vi "PathPlanner_Cmd_AutoLTVUnicycleExecute.vi"(5 "PathPlanner_Cmd_FollowLTVUnicycleConfig":T18={"ControlPastEnd_Sec"=3.0, "Trigger Events"=TRUE, "LTV_Unicycle_Ctrl_Model"={"Max linear ctrl effort M/S"=2.0, "Max angular ctrl effort Rad/S"=0.7, "Max Heading Meas Tol Rad"=2.0, "Max X Pos Meas Tol M"=0.7, "Max Y Pos Meas Tol M"=0.7, "Max Linear Vel M/S"=2.0}, "X Tolerance M"=0.0762, "Y Tolerance M"=0.0762, "Rotation Tolerance DEG"=0.0872665, "Track Width Meters"=1.0, "Max Speed M/S"=4.0, "Period"=0.02} {"LTV_Unicycle_Ctrl_Model"."Max Linear Vel M/S" format="%#_13g"; "LTV_Unicycle_Ctrl_Model"."Max Y Pos Meas Tol M" format="%#_13g"; "LTV_Unicycle_Ctrl_Model"."Max X Pos Meas Tol M" format="%#_13g"; "LTV_Unicycle_Ctrl_Model"."Max Heading Meas Tol Rad" format="%#_13g"; "LTV_Unicycle_Ctrl_Model"."Max angular ctrl effort Rad/S" format="%#_13g"; "LTV_Unicycle_Ctrl_Model"."Max linear ctrl effort M/S" format="%#_13g"}, 6 "PassthroughTime_SEC":dbl=-1.0, 7 "PathPlanner_Cmd_AutoConfig":T3 {"Paths"."IdealStartingState"."Rotation"."SIN" format="%13.4f"; "Paths"."IdealStartingState"."Rotation"."COS" format="%13.4f"; "Paths"."IdealStartingState"."Rotation"."VALUE" format="%13.4f"; "Paths"."PointTowardsZones"."TargetPosition"."Y" format="%14.3f"; "Paths"."PointTowardsZones"."TargetPosition"."X" format="%14.3f"; "Paths"."PointTowardsZones"."RotationOffset"."SIN" format="%13.4f"; "Paths"."PointTowardsZones"."RotationOffset"."COS" format="%13.4f"; "Paths"."PointTowardsZones"."RotationOffset"."VALUE" format="%13.4f"; "Paths"."Waypoints"."nextControl"."Y" format="%14.3f"; "Paths"."Waypoints"."nextControl"."X" format="%14.3f"; "Paths"."Waypoints"."anchor"."Y" format="%14.3f"; "Paths"."Waypoints"."anchor"."X" format="%14.3f"; "Paths"."Waypoints"."prevControl"."Y" format="%14.3f"; "Paths"."Waypoints"."prevControl"."X" format="%14.3f"; "Paths"."AllPoints"."RotationTarget"."rotation"."SIN" format="%13.4f"; "Paths"."AllPoints"."RotationTarget"."rotation"."COS" format="%13.4f"; "Paths"."AllPoints"."RotationTarget"."rotation"."VALUE" format="%13.4f"; "Paths"."AllPoints"."Position"."Y" format="%14.3f"; "Paths"."AllPoints"."Position"."X" format="%14.3f"; "Paths"."GoalEndState"."Rotation"."SIN" format="%13.4f"; "Paths"."GoalEndState"."Rotation"."COS" format="%13.4f"; "Paths"."GoalEndState"."Rotation"."VALUE" format="%13.4f"; "Paths"."RotationTargets"."rotation"."SIN" format="%13.4f"; "Paths"."RotationTargets"."rotation"."COS" format="%13.4f"; "Paths"."RotationTargets"."rotation"."VALUE" format="%13.4f"}, 8 "Enabled":bool=TRUE, 9 "Reset":bool, 10 "CurrentChassisSpeeds":T2 {"vOmega" format="%10.3f"; "vY" format="%10.3f"; "vX" format="%10.3f"}, 11 "Current Pose SI":T20={"TRANSLATION"={"X"=0.0, "Y"=0.0}, "ROTATION"={"VALUE"=0.0, "COS"=1.0, "SIN"=0.0}} {"ROTATION"."SIN" format="%13.4f"; "ROTATION"."COS" format="%13.4f"; "ROTATION"."VALUE" format="%13.4f"; "TRANSLATION"."Y" format="%14.3f"; "TRANSLATION"."X" format="%14.3f"}) -> (0 "Position Error M":dbl, 1 "Complete":bool, 2 "At Reference":bool, 3 "Left Right Speed Dmds":T1)   [LabVIEW 2019, in "PathPlanner24.lvlib"]
doc: "DOCUMENTATION IS NOT COMPLETE.\n \nCalculates the next output of the path following controller for holonomic drive robots. This wraps a Holonomic Drive Control function with the particulars needed to follow a PathPlanner trajectory.\n\nInputs:\n - PathPlanner_Holonomic_Ctrl_Pack_Tuning - cluster - The tuning paraameters for the holonomic drive controller. These are static. They should not be changed after the first call to this function.\n - CurrentPoseSi - pose2d - The current pose calculated by odometry or pose estimation. The pose can be absolute or relative depending on what type of trajectory is being followed.\n - PathPlannerState - cluster - The path palnner trajectory state containing the desired position and velocities of the robot.\n - Reset - boolean - When TRUE the holonomic drive controller is reset. This should be set to TRUE for the first execution of a trajectory.\n - Enabled - boolean - When TRUE, closed loop control is enabled. (Optional. Default: TRUE)\n - Period - double - The loop period in seconds for this controller. (Optional. Default: 0.020)\n\nOutputs:\n - CalcChassisSpeed - cluster - The desired chassis speed in SI units.\n - AtReference - boolean - TRUE if the robots position is within the defined tolerance.\n - PositionError - pose2d - Position error in SI units. How far the robot is away from the desired trajectory position.\n - out_Holonomic_Drive_Ctrl - THe current holonomic drive controller data cluster. This is mainly for diagnostic purposes."
uses:
  <vilib>/Rock Robotics/WPI/ThirdParty/JAS_Junk/TrajLib/TypeDef/POSE2D.ctl
  <vilib>/Rock Robotics/WPI/ThirdParty/JAS_Junk/TrajLib/TypeDef/TRANSLATION2D.ctl
  <vilib>/Rock Robotics/WPI/ThirdParty/JAS_Junk/TrajLib/TypeDef/ROTATION2D.ctl
  TypeDef/PathPlannerCmdPathPlannerAutoConfig.ctl
  TypeDef/PathPlannerCommandUtil.ctl
  ENum/PathPlanner_CommandUtilType_ENUM.ctl
  TypeDef/PathPlannerPath.ctl
  TypeDef/PathPlannerRotationTarget.ctl
  TypeDef/PathPlannerConstraintsZone.ctl
  TypeDef/PathPlannerPathConstraints.ctl
  TypeDef/PathPlannerEventMarker.ctl
  TypeDef/PathPlannerGoalEndState.ctl
  TypeDef/PathPlannerPathPoint.ctl
  TypeDef/PathPlannerWaypoint.ctl
  TypeDef/PathPlannerPointTowardsZone.ctl
  TypeDef/PathPlannerIdealStartingState.ctl
  <vilib>/Rock Robotics/WPI/ThirdParty/JAS_Junk/TrajLib/TypeDef/CHASSIS_SPEEDS.ctl
  <vilib>/Utility/semaphor.llb/Obtain Semaphore Reference.vi
  <vilib>/Rock Robotics/WPI/ThirdParty/JAS_Junk/TrajLib/Timer_Reset.vi
  PathPlanner24.lvlib
  <vilib>/Rock Robotics/WPI/ThirdParty/JAS_Junk/TrajLib/Trajectory_Library.lvlib
  <vilib>/Rock Robotics/WPI/ThirdParty/JAS_Junk/TrajLib/TypeDef/LTV_UNICYCLE_CONTROLLER_MODEL_PARAMS.CTL
  TypeDef/PathPlannerCmdFollowLTVUnicycleConfig.ctl
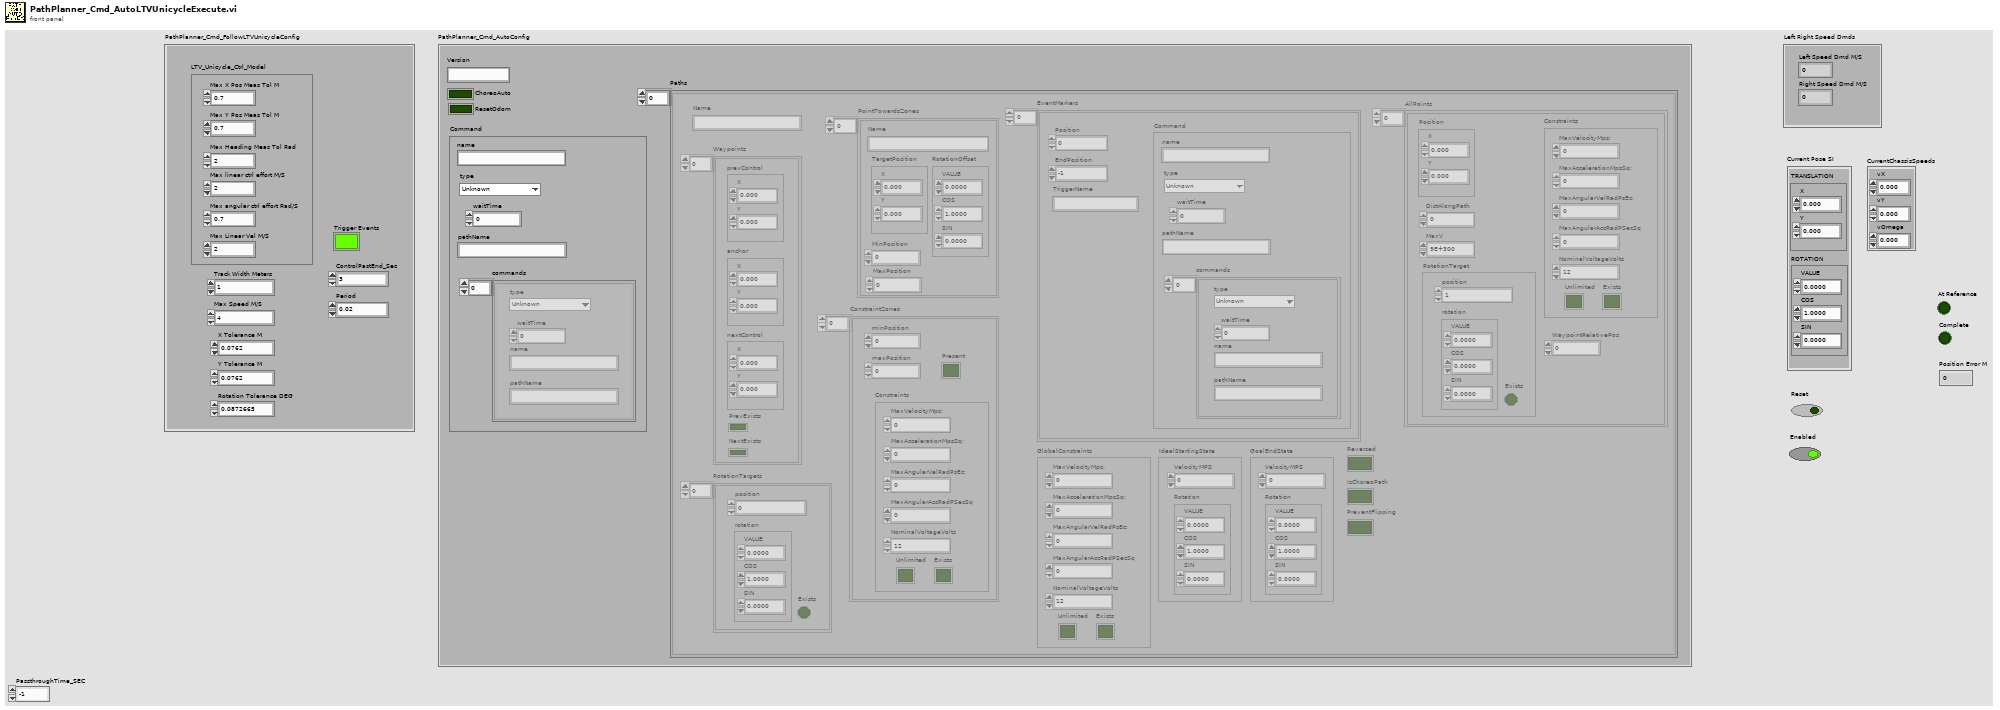
[diagram p1: front panel]
types:
  T1 = cluster{"Left Speed Dmd M/S":dbl, "Right Speed Dmd M/S":dbl}
  T2 = typedef "Trajectory_Library.lvlib/CHASSIS_SPEEDS.ctl" = cluster{"vX":dbl, "vY":dbl, "vOmega":dbl}
  T3 = typedef "PathPlanner24.lvlib/PathPlannerCmdPathPlannerAutoConfig.ctl" = cluster{"Command":T4, "ChoreoAuto":bool, "Version":string, "ResetOdom":bool, "Paths":T6[]}
  T4 = typedef "PathPlanner24.lvlib/PathPlannerCommandUtil.ctl" = cluster{"waitTime":dbl, "name":string, "pathName":string, "commands":cluster{"type":T5, "waitTime":dbl, "name":string, "pathName":string}[], "type":T5}
  T5 = typedef "PathPlanner24.lvlib/PathPlanner_CommandUtilType_ENUM.ctl" = enum16{"Unknown", "Wait", "Named", "Path", "Sequential", "Parallel", "Race", "Deadline"}
  T6 = typedef "PathPlanner24.lvlib/PathPlannerPath.ctl" = cluster{"Reversed":bool, "RotationTargets":T7[], "ConstraintZones":T9[], "EventMarkers":T11[], "GlobalConstraints":T10, "GoalEndState":T12, "AllPoints":T13[], "Name":string, "Waypoints":T15[], "PointTowardsZones":T16[], "IdealStartingState":T17, "IsChoreoPath":bool, "PreventFlipping":bool}
  T7 = typedef "PathPlanner24.lvlib/PathPlannerRotationTarget.ctl" = cluster{"position":dbl, "rotation":T8, "Exists":bool}
  T8 = typedef "Trajectory_Library.lvlib/ROTATION2D.ctl" = cluster{"VALUE":dbl, "COS":dbl, "SIN":dbl}
  T9 = typedef "PathPlanner24.lvlib/PathPlannerConstraintsZone.ctl" = cluster{"minPosition":dbl, "maxPosition":dbl, "Constraints":T10, "Present":bool}
  T10 = typedef "PathPlanner24.lvlib/PathPlannerPathConstraints.ctl" = cluster{"MaxVelocityMps;":dbl, "MaxAccelerationMpsSq;":dbl, "MaxAngularVelRadPsEc;":dbl, "MaxAngularAccRadPSecSq":dbl, "Exists":bool, "Unlimited":bool, "NominalVoltageVolts":dbl}
  T11 = typedef "PathPlanner24.lvlib/PathPlannerEventMarker.ctl" = cluster{"Position":dbl, "Command":T4, "TriggerName":string, "EndPosition":dbl}
  T12 = typedef "PathPlanner24.lvlib/PathPlannerGoalEndState.ctl" = cluster{"VelocityMPS":dbl, "Rotation":T8}
  T13 = typedef "PathPlanner24.lvlib/PathPlannerPathPoint.ctl" = cluster{"Position":T14, "DistAlongPath":dbl, "MaxV":dbl, "Constraints":T10, "RotationTarget":T7, "WaypointRelativePos":dbl}
  T14 = typedef "Trajectory_Library.lvlib/TRANSLATION2D.ctl" = cluster{"X":dbl, "Y":dbl}
  T15 = typedef "PathPlanner24.lvlib/PathPlannerWaypoint.ctl" = cluster{"prevControl":T14, "anchor":T14, "nextControl":T14, "PrevExists":bool, "NextExists":bool}
  T16 = typedef "PathPlanner24.lvlib/PathPlannerPointTowardsZone.ctl" = cluster{"RotationOffset":T8, "Name":string, "TargetPosition":T14, "MinPosition":dbl, "MaxPosition":dbl}
  T17 = typedef "PathPlanner24.lvlib/PathPlannerIdealStartingState.ctl" = cluster{"VelocityMPS":dbl, "Rotation":T8}
  T18 = typedef "PathPlanner24.lvlib/PathPlannerCmdFollowLTVUnicycleConfig.ctl" = cluster{"ControlPastEnd_Sec":dbl, "Trigger Events":bool, "LTV_Unicycle_Ctrl_Model":T19, "X Tolerance M":dbl, "Y Tolerance M":dbl, "Rotation Tolerance DEG":dbl, "Track Width Meters":dbl, "Max Speed M/S":dbl, "Period":dbl}
  T19 = typedef "Trajectory_Library.lvlib/LTV_UNICYCLE_CONTROLLER_MODEL_PARAMS.CTL" = cluster{"Max linear ctrl effort M/S":dbl, "Max angular ctrl effort Rad/S":dbl, "Max Heading Meas Tol Rad":dbl, "Max X Pos Meas Tol M":dbl, "Max Y Pos Meas Tol M":dbl, "Max Linear Vel M/S":dbl}
  T20 = typedef "Trajectory_Library.lvlib/POSE2D.ctl" = cluster{"TRANSLATION":T14, "ROTATION":T8}
  T21 = typedef "Trajectory_Library.lvlib/TIMER.ctl" = cluster{"StartTime":dbl, "Accumulated TIme":dbl, "Running":bool, "semaphore":T22}
  T22 = typedef "Semaphore RefNum" = refnum<k1>
  T23 = cluster{"type":T5, "waitTime":dbl, "name":string, "pathName":string}[]
  T24 = cluster{"type":T5, "waitTime":dbl, "name":string, "pathName":string}
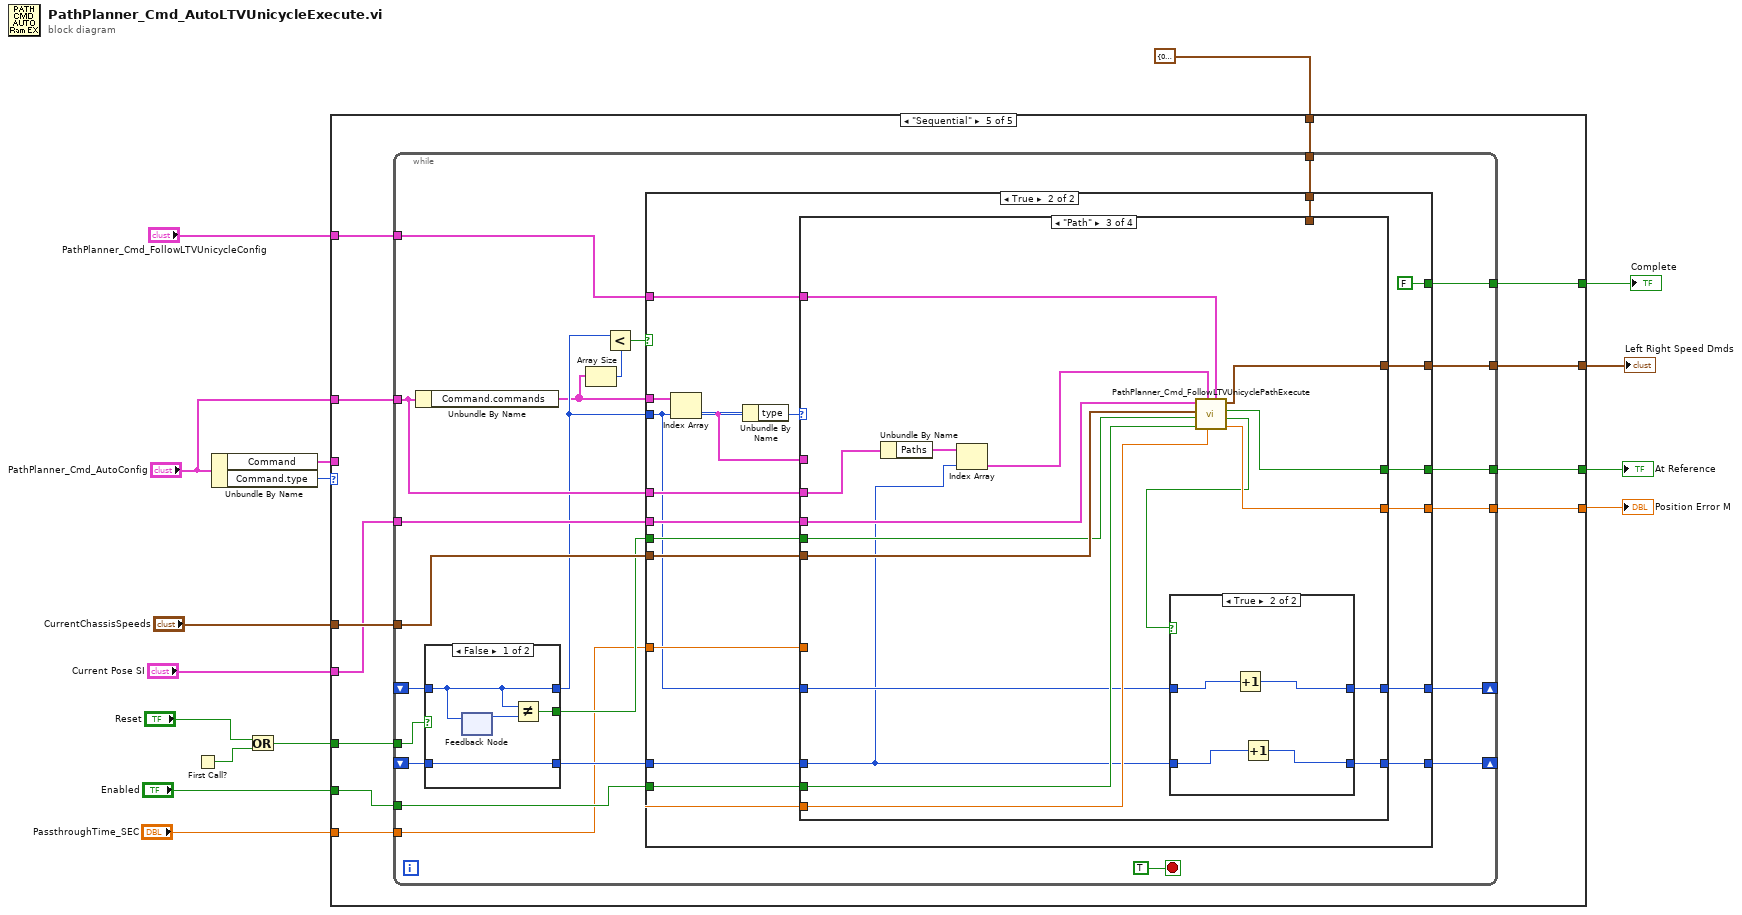
[diagram p0: block diagram]
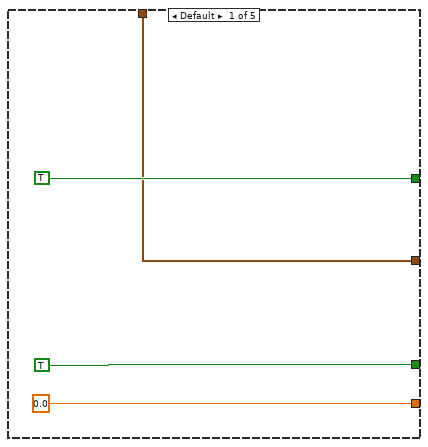
[diagram p2: hidden frame]
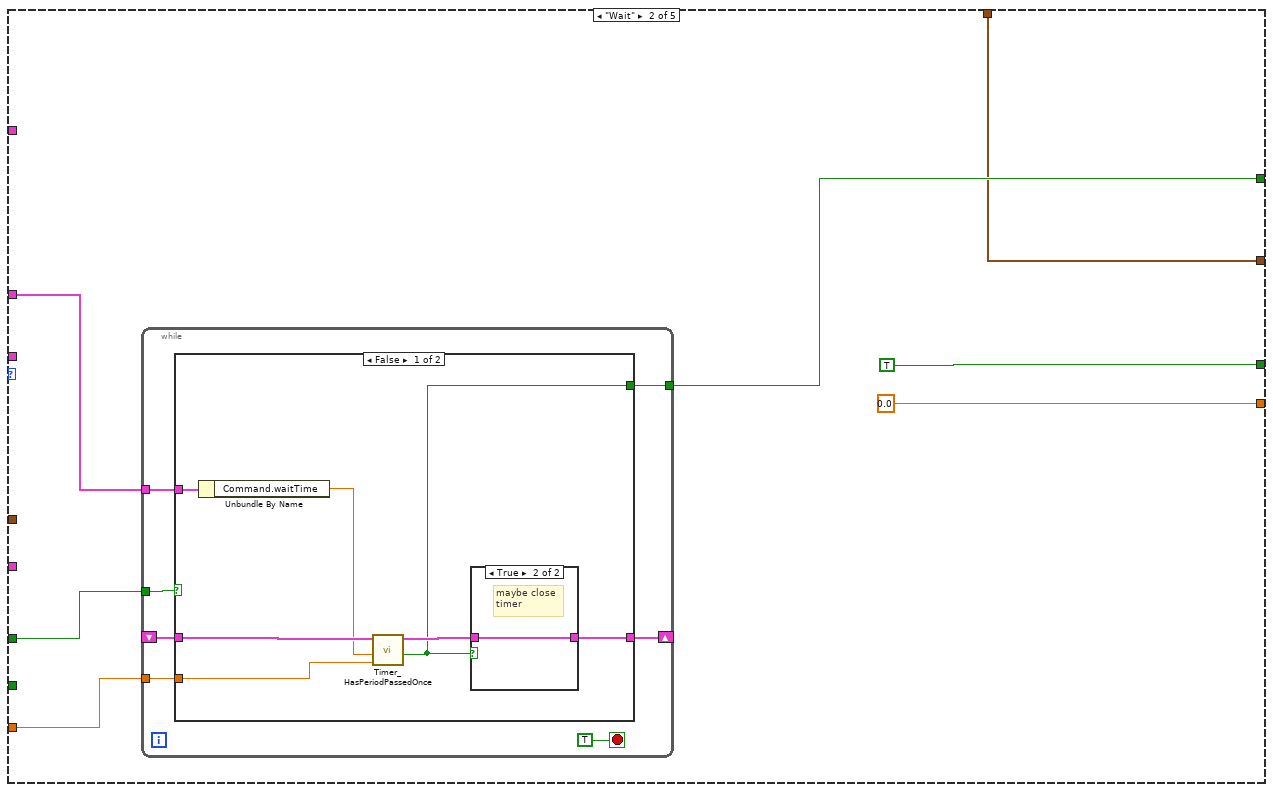
[diagram p3: hidden frame]
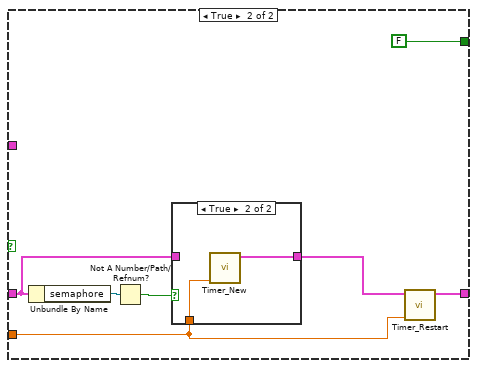
[diagram p5: hidden frame]
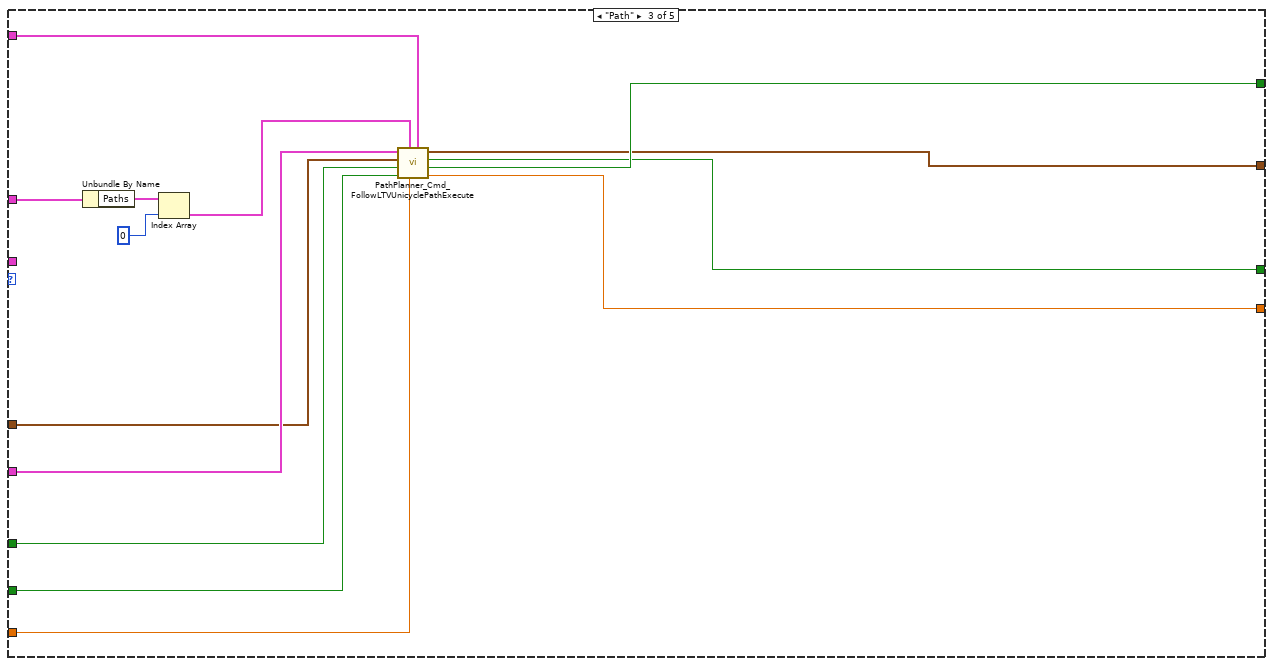
[diagram p7: hidden frame]
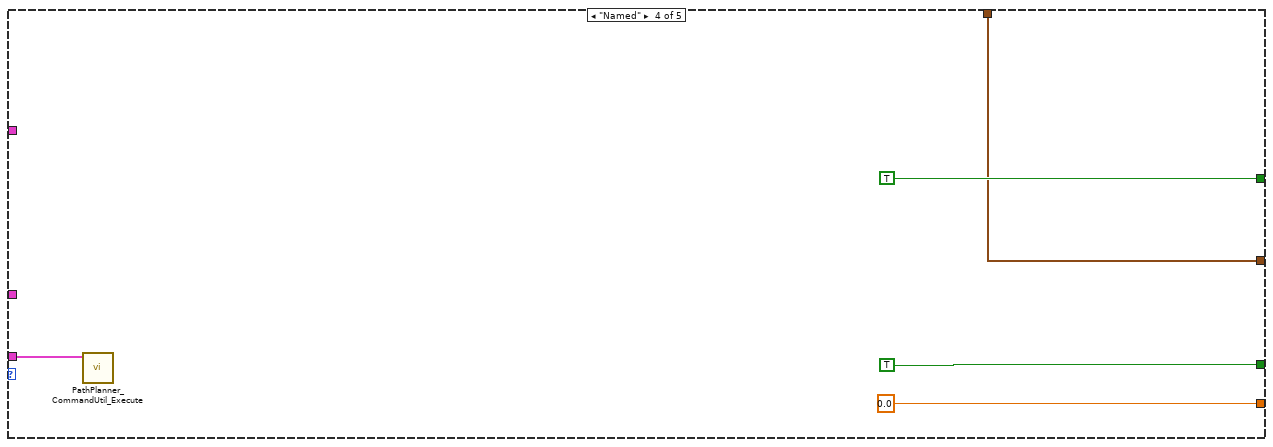
[diagram p8: hidden frame]
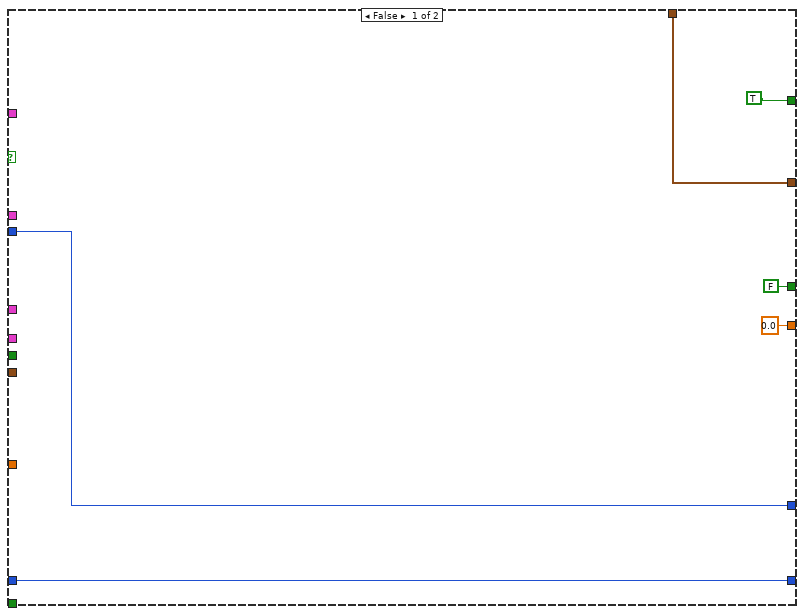
[diagram p9: hidden frame]
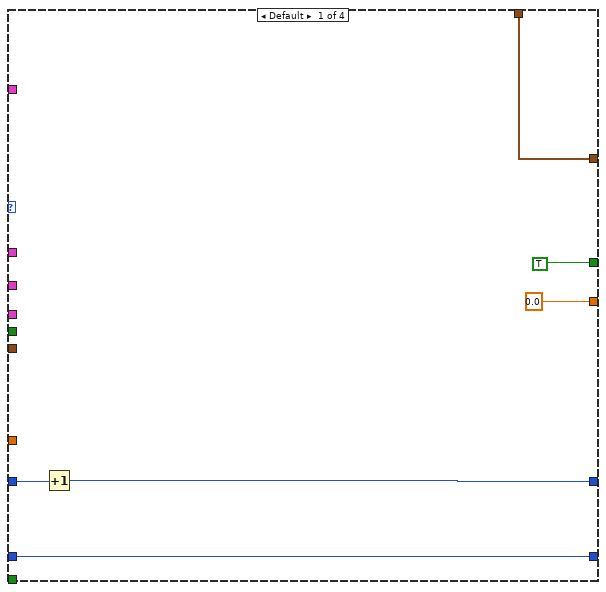
[diagram p10: hidden frame]
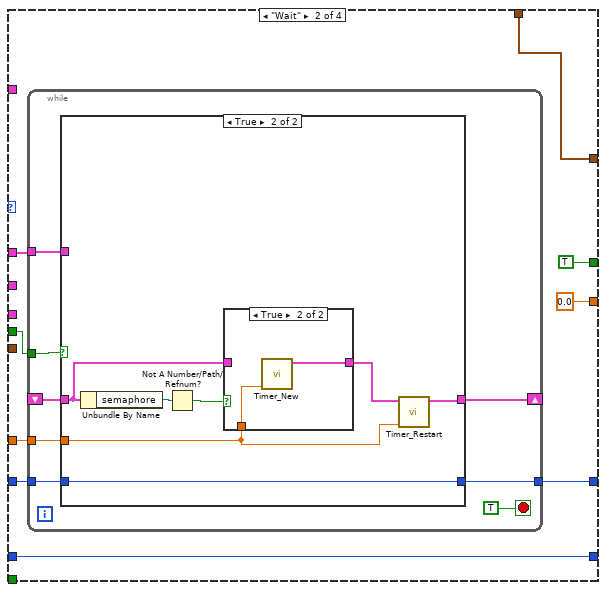
[diagram p11: hidden frame]
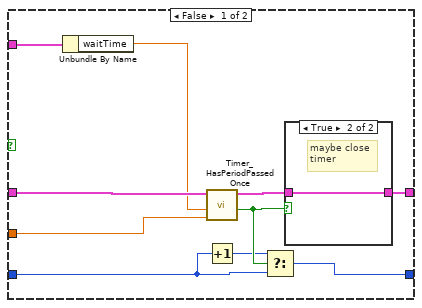
[diagram p12: hidden frame]
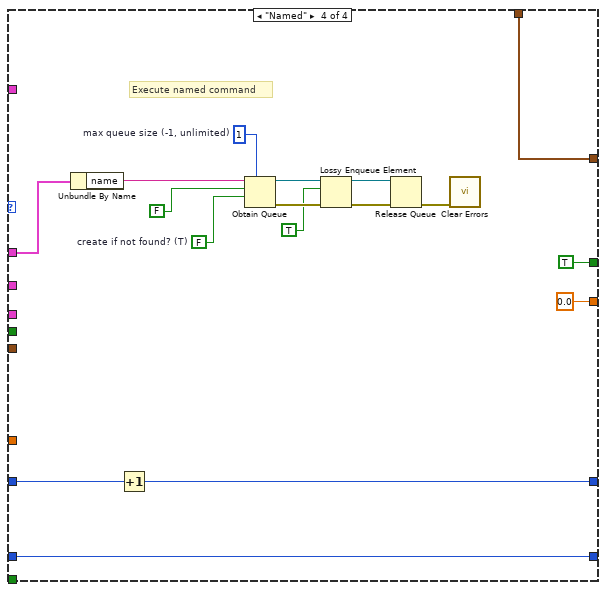
[diagram p16: hidden frame]
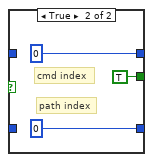
[diagram p17: hidden frame]
diagram:
  n1 = First Call?() -> (First Call?: T/F=w15:bool)
  n2 = Unbundle By Name("PathPlanner_Cmd_AutoConfig") -> ("Command"=w13:T4, "Command.type"=w14:T5)
  n3 = Or(x="Reset", y=w15) -> (x .or. y?=w8:bool)
  n4 = case shown="\"Sequential\"" w14 {
    tunnel: w13 -> [_ _ _ w72 _]
    tunnel: "PathPlanner_Cmd_AutoConfig" -> [_ w25 w67 _ w83]
    tunnel: "PathPlanner_Cmd_FollowLTVUnicycleConfig" -> [_ _ w63 _ w77]
    tunnel: "Current Pose SI" -> [_ _ w62 _ w76]
    tunnel: "CurrentChassisSpeeds" -> [_ _ w61 _ w82]
    tunnel: w8 -> [_ w27 w60 _ w84]
    tunnel: "Enabled" -> [_ _ w59 _ w75]
    tunnel: "PassthroughTime_SEC" -> [_ w26 w58 _ w79]
    tunnel: [0.0 ("Position Error M") 0.0 ("Position Error M") w57 0.0 ("Position Error M") w80] -> w5
    tunnel: [TRUE ("Complete") w24 w56 TRUE ("Complete") w74] -> w4
    tunnel: [TRUE ("At Reference") TRUE ("At Reference") w55 TRUE ("At Reference") w81] -> w3
    tunnel: T1 {"Left Speed Dmd M/S"=0.0, "Right Speed Dmd M/S"=0.0} ("Left Right Speed Dmds") -> [w17 w21 _ w68 w78]
    tunnel: [w17 w21 w54 w68 w73] -> w2
    frame Default {
    }
    frame "Wait" {
      n5 = while {
        tunnel: w27 -> [w34]
        tunnel: w26 -> [w33]
        shift-right: [w32] -> _
        shift-left: _ -> [w31]
        tunnel: w25 -> [w30]
        tunnel: [w28] -> w24
        stop <- TRUE stop-if-true
        n6 = case shown="False" w34 {
          tunnel: w33 -> [w40 w49]
          tunnel: [w36 w48] -> w32
          tunnel: w31 -> [w41 w44]
          tunnel: w30 -> [w39 _]
          tunnel: [w35 FALSE ("Expired")] -> w28
          frame False {
            n7 = Unbundle By Name(w39) -> ("Command.waitTime"=w38:dbl)
            n8 = call <vilib>:"Timer_HasPeriodPassedOnce.vi"("Pass_Through_Time"=w40, "Period"=w38, "in Timer"=w41) -> ("Expired"=w35:bool, "out Timer"=w37:T21)  [unwired: 6 in, 1 out]
            n9 = case shown="True" w35 {
              tunnel: w37 -> [w42 w43]
              tunnel: [w42 w43] -> w36
              frame False {
              }
              frame True {
                # "maybe close\ntimer"
              }
            }
          }
          frame True {
            n10 = Unbundle By Name(w44) -> ("semaphore"=w45:T22)
            n11 = Not A Number/Path/Refnum?(number/path/refnum=w45) -> (NaN/Path/Refnum?=w46:bool)
            n12 = case shown="True" w46 {
              tunnel: [w51 w53] -> w50
              tunnel: w49 -> [_ w52]
              tunnel: w44 -> [w51 _]
              frame False {
              }
              frame True {
                n13 = call <vilib>:"Timer_New.vi"("Pass_Through_Time"=w52) -> ("TIMER"=w53:T21)  [unwired: 10 in]
              }
            }
            n14 = call <vilib>:"Timer_Restart.vi"("Pass_Through_Time"=w49, "in Timer"=w50) -> ("out Timer"=w48:T21)  [unwired: 9 in]
          }
        }
      }
    }
    frame "Path" {
      n15 = Unbundle By Name(w67) -> ("Paths"=w66:T6[])
      n16 = Index Array(array=w66, index=0) -> (element=w64:T6)
      n17 = call "PathPlanner_Cmd_FollowLTVUnicyclePathExecute.vi"("PathPlanner_Cmd_FollowLTVUnicycleConfig"=w63, "PassthroughTime_SEC"=w58, "PathPlannerPath"=w64, "Enabled"=w59, "Reset"=w60, "CurrentChassisSpeeds"=w61, "Current Pose SI"=w62) -> ("Position Error M"=w57:dbl, "Complete"=w56:bool, "At Reference"=w55:bool, "Left Right Speed Dmds"=w54:T1)  [unwired: 1 out]
    }
    frame "Named" {
      n18 = call "PathPlanner_CommandUtil_Execute.vi"("Command"=w72) -> ()  [unwired: 11 in]
    }
    frame "Sequential" {
      n19 = while {
        tunnel: w84 -> [w103]
        tunnel: w83 -> [w98]
        tunnel: w82 -> [w106]
        tunnel: [w105] -> w81
        tunnel: [w104] -> w80
        tunnel: w79 -> [w93]
        shift-right: [w92] -> _
        shift-left: _ -> [w102]
        shift-right: [w91] -> _
        shift-left: _ -> [w101]
        tunnel: w78 -> [w99]
        tunnel: w77 -> [w96]
        tunnel: w76 -> [w95]
        tunnel: w75 -> [w94]
        tunnel: [w86] -> w74
        tunnel: [w85] -> w73
        stop <- TRUE stop-if-true
        n20 = Unbundle By Name(w98) -> ("Command.commands"=w88:T23)
        n21 = case shown="False" w103 {
          tunnel: [w218 0] -> w90
          tunnel: [w220 0] -> w97
          tunnel: w102 -> [w218 _]
          tunnel: w101 -> [w220 _]
          tunnel: [w221 TRUE] -> w100
          frame False {
            n22 = feedback-in #1(w218) -> ()
            n23 = feedback #1() -> (w219:i32)  [unwired: 1 in]
            n24 = Not Equal?(x=w218, y=w219) -> (x != y?=w221:bool)
          }
          frame True {
            # "path index"
            # "cmd index"
          }
        }
        n25 = Array Size(array=w88) -> (size(s)=w89:i32)
        n26 = Less?(x=w90, y=w89) -> (x < y?=w87:bool)
        n27 = case shown="True" w87 {
          tunnel: w106 -> [_ w132]
          tunnel: [FALSE ("At Reference") w131] -> w105
          tunnel: [0.0 ("Position Error M") w130] -> w104
          tunnel: w88 -> [_ w129]
          tunnel: w100 -> [_ w127]
          tunnel: w99 -> [w108 w125]
          tunnel: w98 -> [_ w124]
          tunnel: w97 -> [w109 w123]
          tunnel: w96 -> [_ w122]
          tunnel: w95 -> [_ w121]
          tunnel: w94 -> [_ w120]
          tunnel: w93 -> [_ w119]
          tunnel: w90 -> [w110 w115]
          tunnel: [w110 w118] -> w92
          tunnel: [w109 w117] -> w91
          tunnel: [TRUE FALSE] -> w86
          tunnel: [w108 w114] -> w85
          frame False {
          }
          frame True {
            n28 = Index Array(array=w129, index=w115) -> (element=w126:T24)
            n29 = Unbundle By Name(w126) -> ("type"=w128:T5)
            n30 = case shown="\"Path\"" w128 {
              tunnel: w132 -> [_ _ w189 _]
              tunnel: [TRUE TRUE ("At Reference") w185 TRUE ("At Reference")] -> w131
              tunnel: [0.0 0.0 ("Position Error M") w184 0.0 ("Position Error M")] -> w130
              tunnel: w119 -> [_ w147 _ _]
              tunnel: w127 -> [_ w146 w188 _]
              tunnel: w126 -> [_ w145 _ w207]
              tunnel: w125 -> [w133 w139 _ w201]
              tunnel: w124 -> [_ _ w192 _]
              tunnel: w123 -> [w134 w144 w181 w202]
              tunnel: w122 -> [_ _ w191 _]
              tunnel: w121 -> [_ _ w190 _]
              tunnel: w120 -> [_ _ w187 _]
              tunnel: w119 -> [_ _ w186 _]
              tunnel: w115 -> [w136 w143 w182 w204]
              tunnel: [w135 w142 w179 w203] -> w118
              tunnel: [w134 w144 w180 w202] -> w117
              tunnel: [w133 w139 w178 w201] -> w114
              frame Default {
                n31 = Increment(x=w136) -> (x+1=w135:i32)
              }
              frame "Wait" {
                n32 = while {
                  tunnel: w146 -> [w155]
                  tunnel: w147 -> [w154]
                  shift-right: [w153] -> _
                  shift-left: _ -> [w152]
                  tunnel: w145 -> [w151]
                  tunnel: w143 -> [w149]
                  tunnel: [w148] -> w142
                  stop <- TRUE stop-if-true
                  n33 = case shown="True" w155 {
                    tunnel: w154 -> [w164 w173]
                    tunnel: [w160 w172] -> w153
                    tunnel: w152 -> [w165 w169]
                    tunnel: w151 -> [w163 _]
                    tunnel: w149 -> [w156 w168]
                    tunnel: [w158 w168] -> w148
                    frame False {
                      n34 = Unbundle By Name(w163) -> ("waitTime"=w162:dbl)
                      n35 = call <vilib>:"Timer_HasPeriodPassedOnce.vi"("Pass_Through_Time"=w164, "Period"=w162, "in Timer"=w165) -> ("Expired"=w159:bool, "out Timer"=w161:T21)  [unwired: 6 in, 1 out]
                      n36 = Increment(x=w156) -> (x+1=w157:i32)
                      n37 = Select(t=w157, s=w159, f=w156) -> (s? t:f=w158:i32)
                      n38 = case shown="True" w159 {
                        tunnel: w161 -> [w166 w167]
                        tunnel: [w166 w167] -> w160
                        frame False {
                        }
                        frame True {
                          # "maybe close\ntimer"
                        }
                      }
                    }
                    frame True {
                      n39 = Unbundle By Name(w169) -> ("semaphore"=w170:T22)
                      n40 = Not A Number/Path/Refnum?(number/path/refnum=w170) -> (NaN/Path/Refnum?=w171:bool)
                      n41 = case shown="True" w171 {
                        tunnel: [w175 w177] -> w174
                        tunnel: w173 -> [_ w176]
                        tunnel: w169 -> [w175 _]
                        frame False {
                        }
                        frame True {
                          n42 = call <vilib>:"Timer_New.vi"("Pass_Through_Time"=w176) -> ("TIMER"=w177:T21)  [unwired: 10 in]
                        }
                      }
                      n43 = call <vilib>:"Timer_Restart.vi"("Pass_Through_Time"=w173, "in Timer"=w174) -> ("out Timer"=w172:T21)  [unwired: 9 in]
                    }
                  }
                }
              }
              frame "Path" {
                n44 = Unbundle By Name(w192) -> ("Paths"=w194:T6[])
                n45 = Index Array(array=w194, index=w181) -> (element=w193:T6)
                n46 = call "PathPlanner_Cmd_FollowLTVUnicyclePathExecute.vi"("PathPlanner_Cmd_FollowLTVUnicycleConfig"=w191, "PassthroughTime_SEC"=w186, "PathPlannerPath"=w193, "Enabled"=w187, "Reset"=w188, "CurrentChassisSpeeds"=w189, "Current Pose SI"=w190) -> ("Position Error M"=w184:dbl, "Complete"=w183:bool, "At Reference"=w185:bool, "Left Right Speed Dmds"=w178:T1)  [unwired: 1 out]
                n47 = case shown="True" w183 {
                  tunnel: w182 -> [w195 w200]
                  tunnel: w181 -> [w196 w198]
                  tunnel: [w196 w197] -> w180
                  tunnel: [w195 w199] -> w179
                  frame False {
                  }
                  frame True {
                    n48 = Increment(x=w200) -> (x+1=w199:i32)
                    n49 = Increment(x=w198) -> (x+1=w197:i32)
                  }
                }
              }
              frame "Named" {
                w213 = FALSE  # create if not found? (T)
                w212 = 1  # max queue size (-1, unlimited)
                # "Execute named command"
                n50 = Unbundle By Name(w207) -> ("name"=w211:string)
                n51 = Increment(x=w204) -> (x+1=w203:i32)
                n52 = Obtain Queue(max queue size (-1, unlimited)=w212, name (unnamed)=w211, element data type=FALSE, create if not found? (T)=w213) -> (queue out=w216:refnum<queue>, error out=w217:errorcluster)  [unwired: 1 in, 1 out]
                n53 = Lossy Enqueue Element(queue=w216, element=TRUE, error in (no error)=w217) -> (queue out=w208:refnum<queue>, error out=w209:errorcluster)  [unwired: 2 out]
                n54 = Release Queue(queue=w208, error in (no error)=w209) -> (error out=w210:errorcluster)  [unwired: 1 in, 2 out]
                n55 = call <vilib>:"Clear Errors.vi"("error in (no error)"=w210) -> ()  [unwired: 5 in, 2 out]
              }
            }
          }
        }
      }
    }
  }
  "At Reference" <- w3
  "Position Error M" <- w5
  "Complete" <- w4
  "Left Right Speed Dmds" <- w2
